vi "Drive Forward.vi"(4 "Time":dbl=1.0, 6 "Speed":dbl=1.0, 11 "error in":errorcluster) -> (3 "error out":errorcluster)   [LabVIEW 2015]
uses:
  References/Refnums.vi
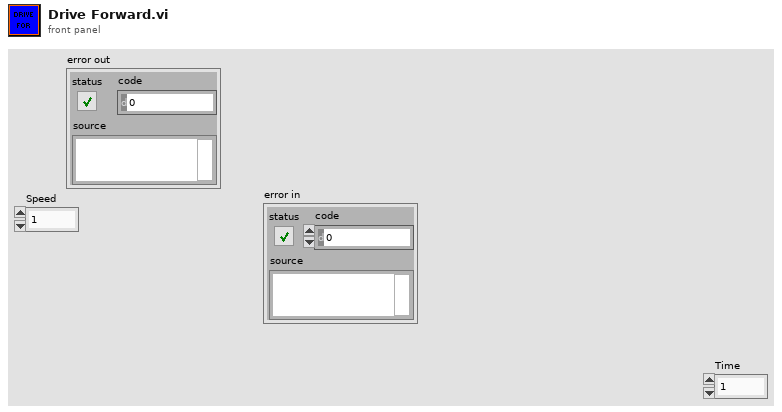
[diagram p1: front panel]
types:
  T1 = typedef "WPI_MotorControlDeviceRef.ctl" = cluster{"DeviceStatus":errorcluster, "Type":T2, "PWM":cluster{"PWM Channel":T3, "DeadBand":T4}, "CAN":cluster{"Device Number":u8, "Control Mode":T5, "Semaphore":T6, "Max Vout":dbl, "TalonSRX Control Mode":T7}, "Invert":bool}
  T2 = typedef "WPI_MotorControlType.ctl" = enum16{"PWM", "CAN", "CANTalonSRX"}
  T3 = typedef "FPGA_DIOPWMChannel.ctl" = enum8{"PWM 0", "PWM 1", "PWM 2", "PWM 3", "PWM 4", "PWM 5", "PWM 6", "PWM 7", "PWM 8", "PWM 9", "PWM MXP 0", "PWM MXP 1", "PWM MXP 2", "PWM MXP 3", "PWM MXP 4", "PWM MXP 5", "PWM MXP 6", "PWM MXP 7", "PWM MXP 8", "PWM MXP 9", "Invalid"}
  T4 = typedef "WPI_PWMDeadband.ctl" = cluster{"Name":string, "maxPositivePwm":i32, "minPositivePwm":i32, "centerPwm":i32, "maxNegativePwm":i32, "minNegativePwm":i32, "angularRange":u16}
  T5 = typedef "WPI_CANJaguar_ControlMode.ctl" = enum8{"Percent VBus", "Current", "Speed", "Position", "Voltage"}
  T6 = typedef "Semaphore RefNum" = refnum<k1>
  T7 = typedef "WPI_CANTalonSRX_APIControlMode.ctl" = enum8{"Percent VBus", "Speed", "Position", "Slave", "Unchanged / Invalid", "Voltage Compensation", "Current", "Motion Profile"}
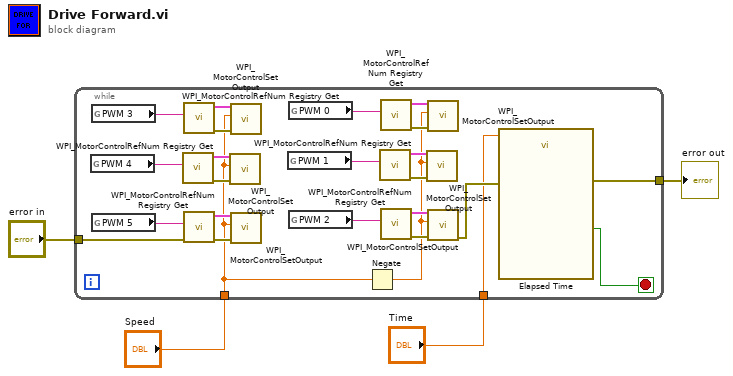
[diagram p0: block diagram]
diagram:
  n1 = while {
    tunnel: [w9] -> w4
    tunnel: "error in" -> [w8]
    tunnel: "Time" -> [w6]
    tunnel: "Speed" -> [w5]
    stop <- w11 stop-if-true
    n2 = global read "Refnums.vi" "PWM 4"() -> (w15:string)
    n3 = global read "Refnums.vi" "PWM 3"() -> (w14:string)
    n4 = global read "Refnums.vi" "PWM 5"() -> (w20:string)
    n5 = call <vilib>:"WPI_MotorControlRefNum Registry Get.vi"("refnum name"=w15) -> ("error out"=w17:errorcluster, "MotorControlDevRef"=w16:T1)  [unwired: 9 in]
    n6 = call <vilib>:"WPI_MotorControlRefNum Registry Get.vi"("refnum name"=w14) -> ("error out"=w12:errorcluster, "MotorControlDevRef"=w13:T1)  [unwired: 9 in]
    n7 = call <vilib>:"WPI_MotorControlRefNum Registry Get.vi"("error in (no error)"=w8, "refnum name"=w20) -> ("error out"=w18:errorcluster, "MotorControlDevRef"=w19:T1)  [unwired: 8 in]
    n8 = call <vilib>:"WPI_MotorControlSetOutput.vi"("error in (no error)"=w17, "Output"=w5, "MotorControlDevRef"=w16) -> ()  [unwired: 6 in, 3 out]
    n9 = call <vilib>:"WPI_MotorControlSetOutput.vi"("error in (no error)"=w12, "Output"=w5, "MotorControlDevRef"=w13) -> ()  [unwired: 6 in, 3 out]
    n10 = call <vilib>:"WPI_MotorControlSetOutput.vi"("error in (no error)"=w18, "Output"=w5, "MotorControlDevRef"=w19) -> ()  [unwired: 6 in, 3 out]
    n11 = global read "Refnums.vi" "PWM 1"() -> (w26:string)
    n12 = global read "Refnums.vi" "PWM 0"() -> (w27:string)
    n13 = global read "Refnums.vi" "PWM 2"() -> (w21:string)
    n14 = Negate(x=w5) -> (-x=w7:dbl)
    n15 = call <vilib>:"WPI_MotorControlRefNum Registry Get.vi"("refnum name"=w26) -> ("error out"=w24:errorcluster, "MotorControlDevRef"=w25:T1)  [unwired: 9 in]
    n16 = call <vilib>:"WPI_MotorControlRefNum Registry Get.vi"("refnum name"=w27) -> ("error out"=w29:errorcluster, "MotorControlDevRef"=w28:T1)  [unwired: 9 in]
    n17 = call <vilib>:"WPI_MotorControlRefNum Registry Get.vi"("refnum name"=w21) -> ("error out"=w23:errorcluster, "MotorControlDevRef"=w22:T1)  [unwired: 9 in]
    n18 = call <vilib>:"WPI_MotorControlSetOutput.vi"("error in (no error)"=w24, "Output"=w7, "MotorControlDevRef"=w25) -> ()  [unwired: 6 in, 3 out]
    n19 = call <vilib>:"WPI_MotorControlSetOutput.vi"("error in (no error)"=w29, "Output"=w7, "MotorControlDevRef"=w28) -> ()  [unwired: 6 in, 3 out]
    n20 = call <vilib>:"WPI_MotorControlSetOutput.vi"("error in (no error)"=w23, "Output"=w7, "MotorControlDevRef"=w22) -> ("error out"=w10:errorcluster)  [unwired: 6 in, 2 out]
    n21 = call "Elapsed Time"("Time Target (s)"=w6, "error in (no error)"=w10) -> ("Time has Elapsed"=w11:bool, "error out"=w9:errorcluster)  [unwired: 10 in, 6 out]
  }
  "error out" <- w4
